vi "BLE_Get_WatcherResponse.vi"(0 ".NET Refnum in":refnum<k24>, 11 "error in (no error)":errorcluster) -> (4 ".NET Refnum out":refnum<k24>, 6 "Watcher Response":string, 8 "Bluetooth Addr":string, 10 "Bluetooth Raw Addr":string, 15 "error out":errorcluster)   [LabVIEW 2020]
uses:
  C:/Users/bharathi.t/Downloads/Bluetooth - Copy/Bluetooth/BLE/BLELib.dll
  BLELib.dll
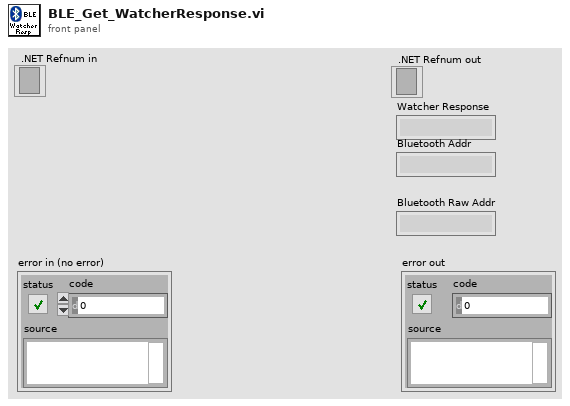
[diagram p1: front panel]
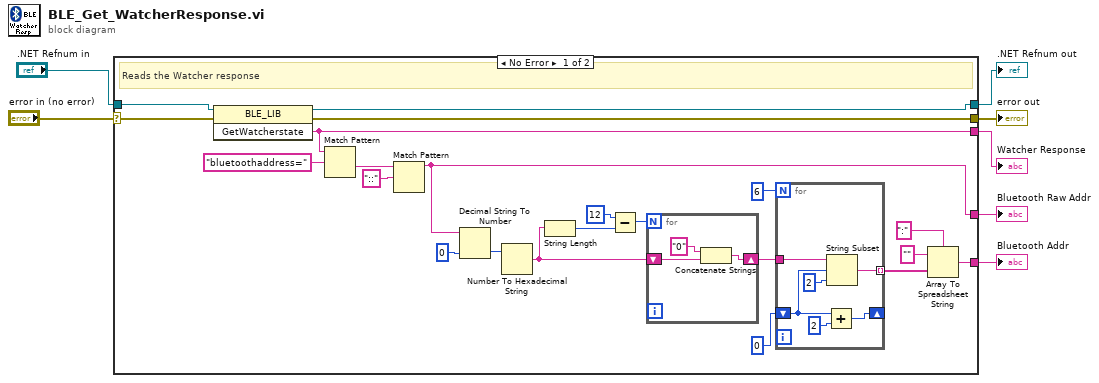
[diagram p0: block diagram]
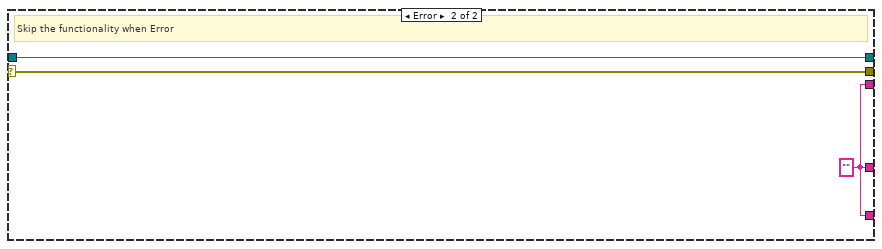
[diagram p2: hidden frame]
diagram:
  n1 = case shown="No Error" "error in (no error)" {
    selector: "error in (no error)" -> [w26 w40]
    tunnel: ".NET Refnum in" -> [w29 w41]
    tunnel: [w28 w40] -> w6
    tunnel: [w27 w41] -> w5
    tunnel: [w16 w39] -> w3
    tunnel: [w8 w39] -> w2
    tunnel: [w9 w39] -> w1
    frame No Error {
      # "Reads the Watcher response"
      n2 = invoke class="BLE_LIB" method="GetWatcherstate"(reference=w29, error in=w26) -> (reference out=w27:refnum<k24>, error out=w28:errorcluster, "GetWatcherstate"=w16:string)  [unwired: 1 in]
      n3 = Match Pattern(string=w16, regular expression="bluetoothaddress=") -> (after substring=w21:string)  [unwired: 1 in, 3 out]
      n4 = Match Pattern(string=w21, regular expression="::") -> (before substring=w9:string)  [unwired: 1 in, 3 out]
      n5 = Decimal String To Number(string=w9, default (0L)=i64 0 ("default (0 I32)")) -> (number=w24:i64)  [unwired: 1 in, 1 out]
      n6 = Number To Hexadecimal String(2:w24) -> (0:w17:string)  [unwired: 1 in]
      n7 = String Length(string=w17) -> (length=w20:i32)
      n8 = Subtract(x=12, y=w20) -> (x-y=w18:i32)
      n9 = for {
        N: w18 -> [_]
        shift-right: [w36] -> w14
        shift-left: w17 -> [w38]
        n10 = Concatenate Strings("0" ("string"), w38) -> (w36:string)
      }
      n11 = for {
        N: 6 -> [_]
        tunnel: w14 -> [w35]
        shift-right: [w31] -> _
        shift-left: 0 ("offset (0)") -> [w33]
        tunnel: [w30] -> w12 mode=indexing
        n12 = Add(x=w33, y=2) -> (x+y=w31:i32)
        n13 = String Subset(string=w35, offset (0)=w33, length (rest)=2 ("length (rest)")) -> (substring=w30:string)
      }
      n14 = Array To Spreadsheet String(delimiter (Tab)=":", array=w12, 3:"" ("format string")) -> (spreadsheet string=w8:string)
    }
    frame Error {
      w39 = "" ("GetWatcherstate")
      # "Skip the functionality when Error"
    }
  }
  "Watcher Response" <- w3
  "error out" <- w6
  ".NET Refnum out" <- w5
  "Bluetooth Addr" <- w2
  "Bluetooth Raw Addr" <- w1
